vi "AD_continu.vi"() -> ()   [LabVIEW 2012]
uses:
  Usb_Daq_V52_Dll.dll
panel:
  in  "过采样":i32 min=0 max=7
  out "Numeric":dbl
  out "Waveform Graph":dynamicdata(graph)
  in  "stop":bool
  in  "start":bool
  in  "采样频率":i32=1000 min=100 max=100000 step=1
  in  "采样个数":i32=1024 min=512 step=512
  in  "放大倍数":i32 min=0 max=1 step=1
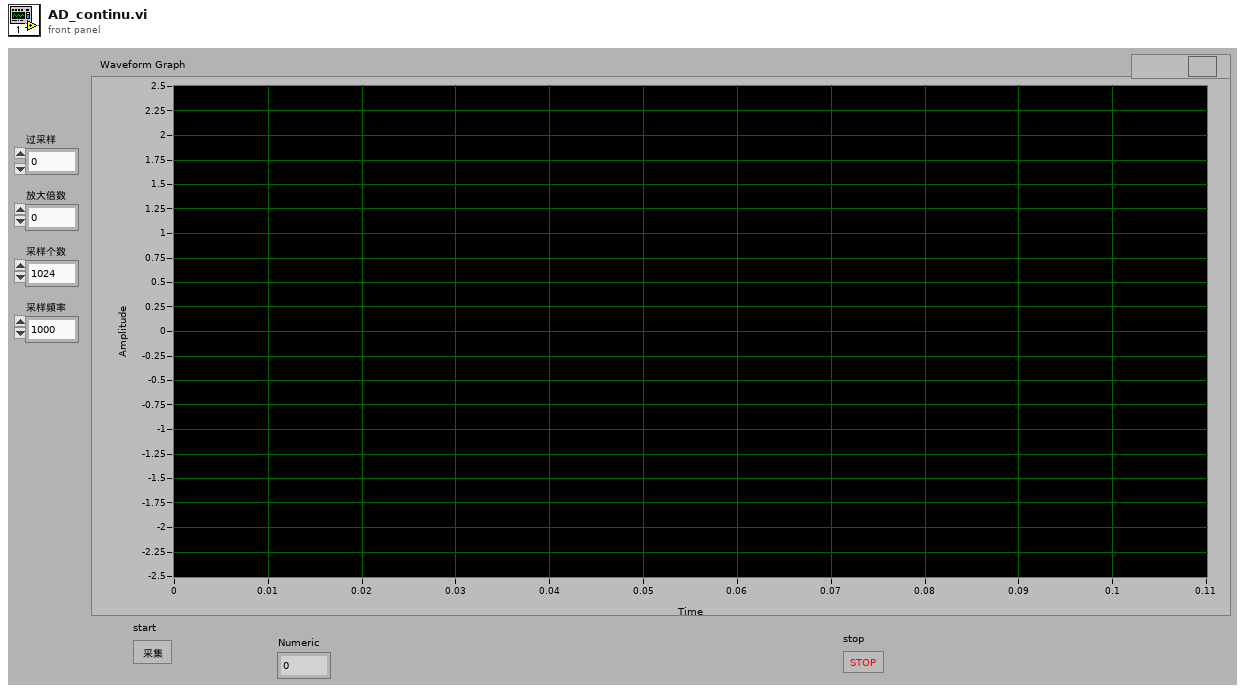
[diagram p1: front panel]
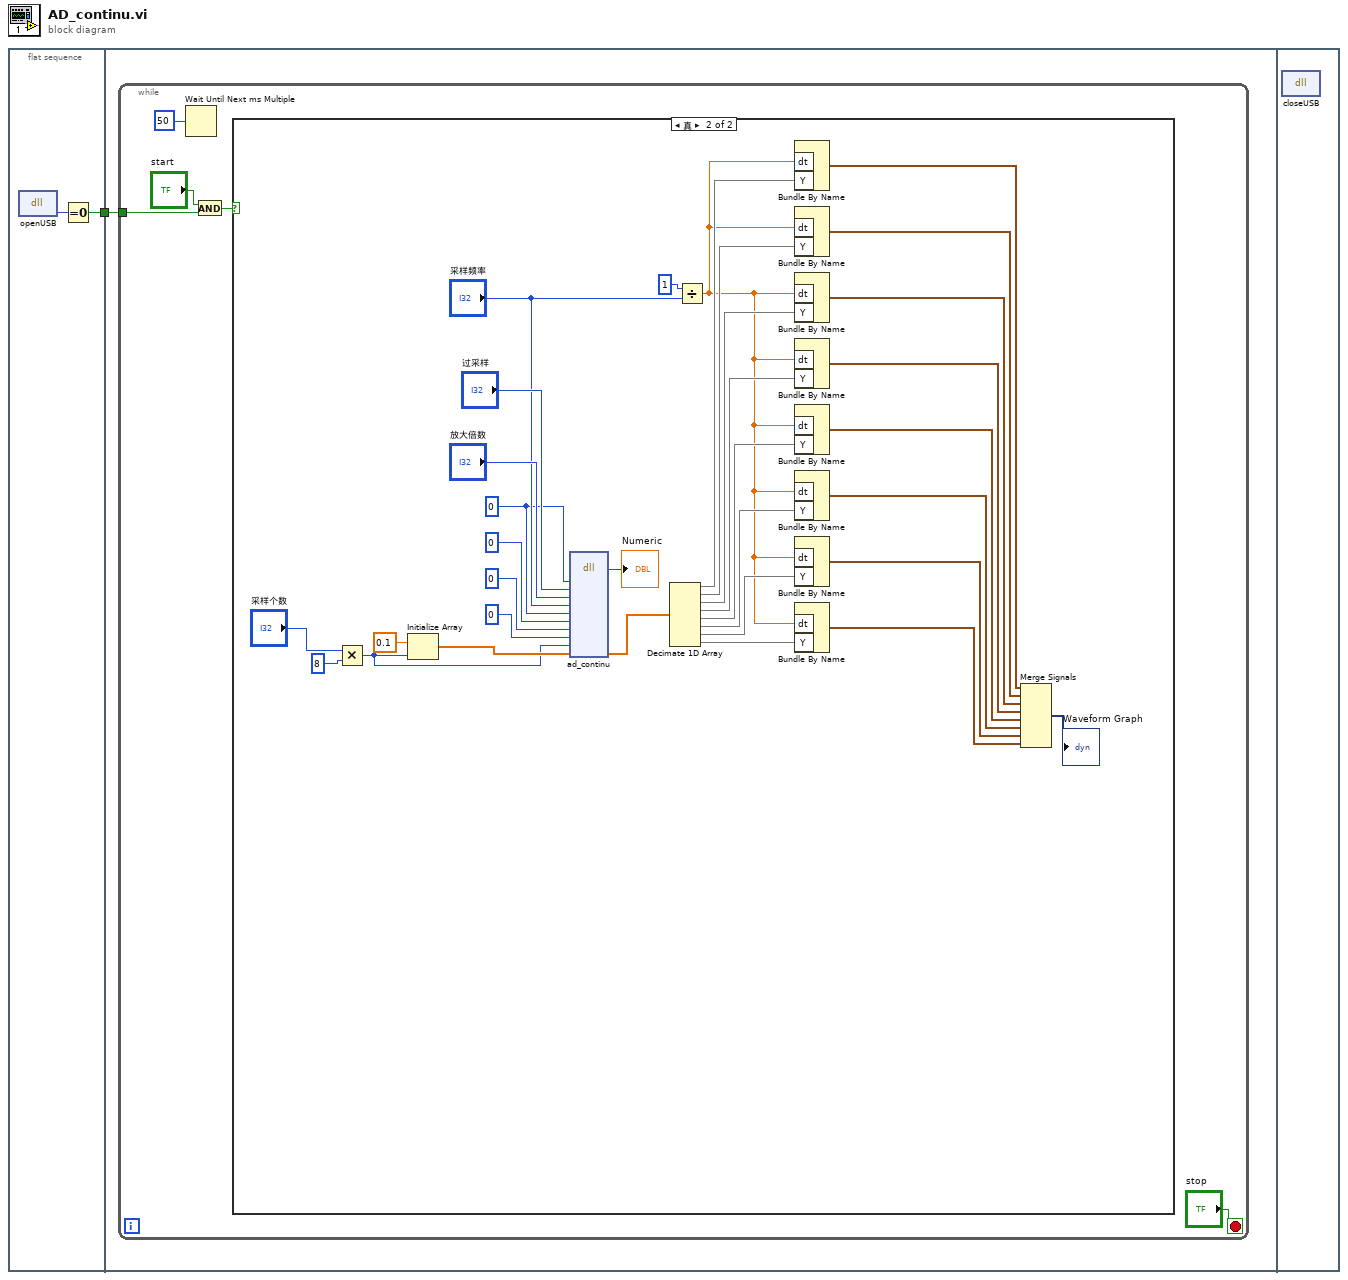
[diagram p0: block diagram]
diagram:
  n1 = flat-sequence {
    tunnel: [w2] -> w1
    tunnel: w1 -> [w4]
    frame #0 {
      n2 = dll-call lib="PTH1labs Ebackup数据采集卡uSB!USB数据采集卡资料HKUSB6203例程labviewUsb_Daq_V52_Dll.dll" fn="openUSB"() -> ("返回类型"=w3:i32)  [unwired: 3 in, 2 out]
      n3 = Equal To 0?(x=w3) -> (x = 0?=w2:bool)
    }
    frame #1 {
      n4 = while {
        tunnel: w4 -> [w5]
        stop <- "stop" stop-if-true
        n5 = Wait Until Next ms Multiple(millisecond multiple=50) -> ()  [unwired: 1 out]
        n6 = And(x="start", y=w5) -> (x .and. y?=w7:bool)
        n7 = case shown="真" w7 {
          frame False {
          }
          frame True {
            w10 = 0
            n8 = Multiply(x="采样个数", y=8) -> (x*y=w11:i32)
            n9 = Initialize Array(0.1, w11) -> (w40:dbl[])
            n10 = dll-call lib="PTH1labs Ebackup数据采集卡uSB!USB数据采集卡资料HKUSB6203例程labviewUsb_Daq_V52_Dll.dll" fn="ad_continu"("dev"=w10, "ad_os"="过采样", "gain"="放大倍数", "Rate_Sample"="采样频率", "trig_sl"=w10, "trig_pol"=0, "clk_sl"=0, "ext_clk_pol"=0, "Num_Sample"=w11, "databuf"=w40) -> ("返回类型"=→"Numeric":i32, "databuf"=w36:sgl[])  [unwired: 11 in, 3 out]
            n11 = Decimate 1D Array(w36) -> (w33:sgl[], w31:sgl[], w30:sgl[], w29:sgl[], w28:sgl[], w27:sgl[], w26:sgl[], w25:sgl[])
            n12 = Divide(x=1, y="采样频率") -> (x/y=w12:dbl)
            n13 = Bundle By Name ("创建波形")("dt"=w12, "Y"=w33) -> (w23:waveform(sgl))  [unwired: 1 in]
            n14 = Bundle By Name ("创建波形")("dt"=w12, "Y"=w31) -> (w22:waveform(sgl))  [unwired: 1 in]
            n15 = Bundle By Name ("创建波形")("dt"=w12, "Y"=w30) -> (w21:waveform(sgl))  [unwired: 1 in]
            n16 = Bundle By Name ("创建波形")("dt"=w12, "Y"=w29) -> (w20:waveform(sgl))  [unwired: 1 in]
            n17 = Bundle By Name ("创建波形")("dt"=w12, "Y"=w28) -> (w19:waveform(sgl))  [unwired: 1 in]
            n18 = Bundle By Name ("创建波形")("dt"=w12, "Y"=w27) -> (w18:waveform(sgl))  [unwired: 1 in]
            n19 = Bundle By Name ("创建波形")("dt"=w12, "Y"=w26) -> (w17:waveform(sgl))  [unwired: 1 in]
            n20 = Bundle By Name ("创建波形")("dt"=w12, "Y"=w25) -> (w13:waveform(sgl))  [unwired: 1 in]
            n21 = Merge Signals(w23, w22, w21, w20, w19, w18, w17, w13) -> (→"Waveform Graph":dynamicdata)
          }
        }
      }
    }
    frame #2 {
      n22 = dll-call lib="PTH1labs Ebackup数据采集卡uSB!USB数据采集卡资料HKUSB6203例程labviewUsb_Daq_V52_Dll.dll" fn="closeUSB"() -> ()  [unwired: 3 in, 3 out]
    }
  }
